vi "Vi Path.vi"(3 "error in":errorcluster, 5 "vi path":path) -> (0 "error out":errorcluster, 1 "vi reference":refnum<vi>, 2 "full path":path)   [LabVIEW 2009]
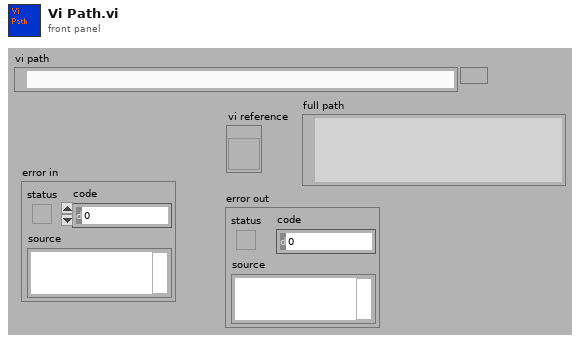
[diagram p1: front panel]
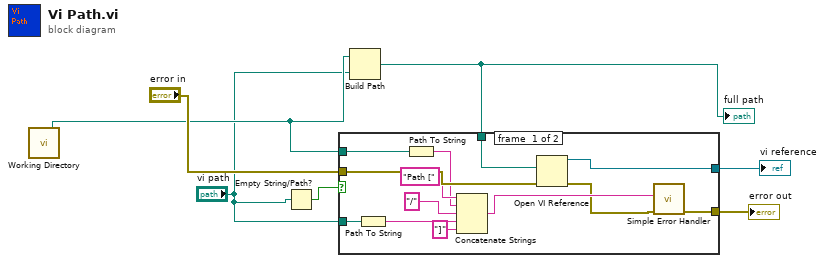
[diagram p0: block diagram]
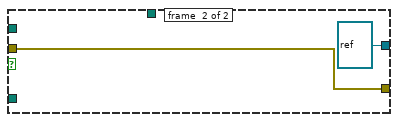
[diagram p2: hidden frame]
diagram:
  n1 = call "Working Directory.vi"() -> ("Path"=w3:path)  [unwired: 1 in]
  n2 = Empty String/Path?(string/path="vi path") -> (empty?=w1:bool)
  n3 = Build Path(base path=w3, name or relative path="vi path") -> (appended path=w7:path)
  "full path" <- w7
  n4 = case shown="True" w1 {
    tunnel: w7 -> [w20 _]
    tunnel: "error in" -> [w19 w21]
    tunnel: [w18 refnum<vi> refnum] -> w5
    tunnel: [w17 w21] -> w4
    tunnel: w3 -> [w15 _]
    tunnel: "vi path" -> [w12 _]
    frame #0 {
      n5 = Path To String(path=w12) -> (string=w11:string)
      n6 = Path To String(path=w15) -> (string=w14:string)
      n7 = Concatenate Strings("Path [" ("string"), w14, "/" ("string"), w11, "]" ("string")) -> (w9:string)
      n8 = Open VI Reference(vi path=w20, error in (no error)=w19) -> (vi reference=w18:refnum<vi>, error out=w8:errorcluster)  [unwired: 4 out]
      n9 = call <vilib>:"Simple Error Handler.vi"("error source (\" \")"=w9, "error in (no error)"=w8) -> ("error out"=w17:errorcluster)  [unwired: 1 in, 6 out]
    }
    frame #1 {
    }
  }
  "error out" <- w4
  "vi reference" <- w5
